vi "svfa_Compute Dual Cross Spectrum Subset.vi"(0 "Windowed signal [X]":waveform(dbl), 1 "processing control":T7(ring), 2 "Spectrum Settings":T10 {"stop frequency" format="%.2f"; "start frequency" format="%.2f"}, 5 "Windowed signal [Y]":waveform(dbl), 7 "window":u16(ring)=1 items=["None "=0, "Hanning"=1, "Hamming"=2, "Blackman-Harris"=3, "Exact Blackman"=4, "Blackman"=5, "Flat Top"=6, "4 Term B-Harris "=7, "7 Term B-Harris"=8, "Low Sidelobe"=9, "Force - Exponential"=10, "Gaussian"=62], 9 "window size":i32, 11 "error in":errorcluster, 12 "averaging parameters":T9={"averaging mode"=enum."No averaging", "weighting mode"=enum."Linear", "number of averages"=10, "linear mode"=enum."Auto restart"}, 13 "spectrum info in":T1={"channel name"="", "description"="", "x-axis units"=0, "spectral info"={"spectrum type"=enum."Power [Magnitude^2]", "linear/dB"=enum."linear", "window"=0, "window size"=0, "FFT size"=0}, "engineering units"=0, "custom label"="", "dB reference [EU]"=0.0, "peak units"=enum."rms", "weighting filter"=0, "spectral density?"=FALSE, "unit label"="", "spectrum skewed?"=FALSE, "complimentary spectrum units"=enum."none"} {"x-axis units" items=["Time (s)"=0, "Frequency-CB (Hz)"=1, "Frequency-CPB (Hz)"=1248, "Frequency-Arbitrary (Hz)"=2357, "Quefrency (s)"=2, "Revolutions (rev)"=3, "Order"=4, "Speed (RPM)"=11, "Speed (rad/s)"=21, "Index"=65535]; "weighting filter" items=["Linear", "A-weighting", "B-weighting", "C-weighting", "ITU-R 468-4", "Dolby", "CCITT", "C-message", "Wb", "Wc", "Wd", "We", "Wf", "Wh", "Wj", "Wk", "Wm", "AES17 20 kHz lowpass", "AES17 40 kHz lowpass", "AES17 20 kHz highpass", "AES17 40 kHz highpass"]; "dB reference [EU]" format="%.2f"; "engineering units" items=["custom..."=0, "V"=1, "A"=21, "C"=30, "pC"=31, "s"=32, "-"=29, "Pa"=2, "N"=20, "g"=3, "m/s^2"=4, "m/s"=5, "m"=6, "mm/s"=12, "mm"=13, "micron/s"=14, "micron"=15, "in/s^2"=7, "in/s"=8, "in"=9, "mil/s"=10, "mil"=11, "rad/s^2"=16, "rad/s"=17, "rad"=18, "deg/s^2"=26, "deg/s"=27, "deg"=28, "RPM"=22, "cycle/s^2"=23, "Hz"=24, "cycle"=25, "strain"=19]; "spectral info"."window" items=["None "=0, "Hanning"=1, "Hamming"=2, "Blackman-Harris"=3, "Exact Blackman"=4, "Blackman"=5, "Flat Top"=6, "4 Term B-Harris "=7, "7 Term B-Harris"=8, "Low Sidelobe"=9, "Force - Exponential"=10, "Gaussian"=62]}) -> (4 "complex spectrum":T8={"f0"=0.0, "df"=1.0, "complex spectrum"=[]} {"complex spectrum" format="%.2f"; "df" format="%.2f"; "f0" format="%.2f"}, 6 "averaging done":bool, 8 "averages completed":dbl format="%.2f", 10 "spectrum info out":T1={"channel name"="", "description"="", "x-axis units"=0, "spectral info"={"spectrum type"=enum."Power [Magnitude^2]", "linear/dB"=enum."linear", "window"=0, "window size"=0, "FFT size"=0}, "engineering units"=0, "custom label"="", "dB reference [EU]"=0.0, "peak units"=enum."rms", "weighting filter"=0, "spectral density?"=FALSE, "unit label"="", "spectrum skewed?"=FALSE, "complimentary spectrum units"=enum."none"} {"x-axis units" items=["Time (s)"=0, "Frequency-CB (Hz)"=1, "Frequency-CPB (Hz)"=1248, "Frequency-Arbitrary (Hz)"=2357, "Quefrency (s)"=2, "Revolutions (rev)"=3, "Order"=4, "Speed (RPM)"=11, "Speed (rad/s)"=21, "Index"=65535]; "weighting filter" items=["Linear", "A-weighting", "B-weighting", "C-weighting", "ITU-R 468-4", "Dolby", "CCITT", "C-message", "Wb", "Wc", "Wd", "We", "Wf", "Wh", "Wj", "Wk", "Wm", "AES17 20 kHz lowpass", "AES17 40 kHz lowpass", "AES17 20 kHz highpass", "AES17 40 kHz highpass"]; "dB reference [EU]" format="%.2f"; "engineering units" items=["custom..."=0, "V"=1, "A"=21, "C"=30, "pC"=31, "s"=32, "-"=29, "Pa"=2, "N"=20, "g"=3, "m/s^2"=4, "m/s"=5, "m"=6, "mm/s"=12, "mm"=13, "micron/s"=14, "micron"=15, "in/s^2"=7, "in/s"=8, "in"=9, "mil/s"=10, "mil"=11, "rad/s^2"=16, "rad/s"=17, "rad"=18, "deg/s^2"=26, "deg/s"=27, "deg"=28, "RPM"=22, "cycle/s^2"=23, "Hz"=24, "cycle"=25, "strain"=19]; "spectral info"."window" items=["None "=0, "Hanning"=1, "Hamming"=2, "Blackman-Harris"=3, "Exact Blackman"=4, "Blackman"=5, "Flat Top"=6, "4 Term B-Harris "=7, "7 Term B-Harris"=8, "Low Sidelobe"=9, "Force - Exponential"=10, "Gaussian"=62]}, 15 "error out":errorcluster)   [LabVIEW 2017]
uses:
  <vilib>/addons/_NISVFA/_Shared subVIs/Controls/svc_Spectrum Info.ctl
  <vilib>/addons/_NISVFA/_Shared subVIs/Controls/svc_X-Axis Units.ctl
  <vilib>/addons/_NISVFA/_Shared subVIs/Controls/svc_Spectrum Type.ctl
  <vilib>/addons/_NISVFA/_Shared subVIs/Controls/svc_Engineering Units Text Ring.ctl
  <vilib>/addons/_NISVFA/_Shared subVIs/Controls/svc_Weighting Filter Text Ring.ctl
  <vilib>/addons/_NISVFA/_Shared subVIs/Controls/svc_Complimentary Spectrum Units.ctl
  <vilib>/addons/_NISVFA/_Shared subVIs/Spectrum Averaging/svfa_Average Spectrum (complex) No State.vi
  <vilib>/addons/_NISVFA/_Shared subVIs/Spectrum Averaging/svfa_Reset Averaging State Info.vi
  <vilib>/addons/_NISVFA/_Shared subVIs/Spectrum Averaging/svfa_Average Array with Avg Checks (complex) No State.vi
  <vilib>/addons/_NISVFA/_Shared subVIs/Spectrum Averaging/svfa_Average Array (complex) No State.vi
  <vilib>/addons/_NISVFA/_Shared subVIs/Spectrum Averaging/svfa_No Average Array (complex).vi
  <vilib>/addons/_NISVFA/_Shared subVIs/Spectrum Averaging/svfa_Average Array (complex).vi
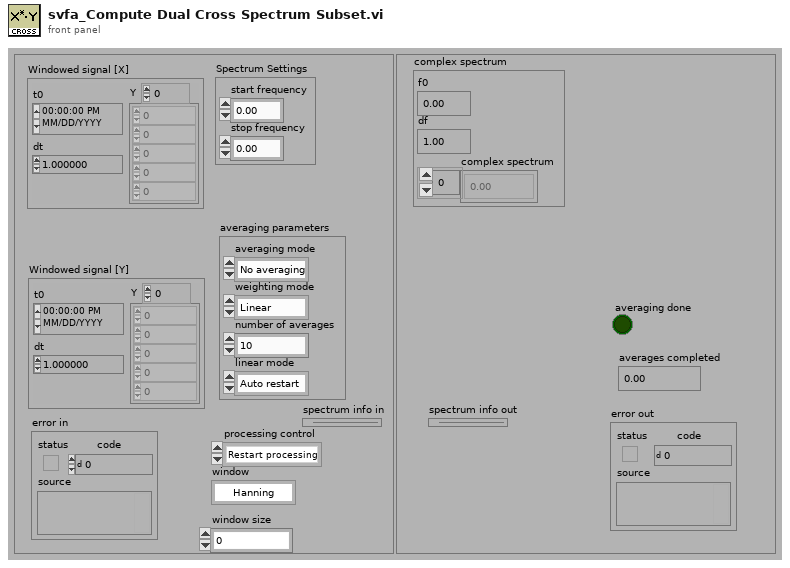
[diagram p1: front panel]
types:
  T1 = typedef "svc_Spectrum Info.ctl" = cluster{"channel name":string, "description":string, "x-axis units":T2, "spectral info":cluster{"spectrum type":T3, "linear/dB":enum16{"linear", "dB"}, "window":u16, "window size":i32, "FFT size":i32}, "engineering units":T4, "custom label":string, "dB reference [EU]":dbl, "peak units":enum16{"rms", "peak", "peak-peak"}, "weighting filter":T5, "spectral density?":bool, "unit label":string, "spectrum skewed?":bool, "complimentary spectrum units":T6}
  T2 = typedef "svc_X-Axis Units.ctl" = u16
  T3 = typedef "svc_Spectrum Type.ctl" = enum16{"FFT Spectrum [complex]", "Amplitude [Magnitude]", "Power [Magnitude^2]", "Cross Spectrum [complex]", "Frequency Response [Complex]"}
  T4 = typedef "svc_Engineering Units Text Ring.ctl" = u16
  T5 = typedef "svc_Weighting Filter Text Ring.ctl" = u16
  T6 = typedef "svc_Complimentary Spectrum Units.ctl" = enum16{"none", "radians", "degrees", "cycles", "imaginary"}
  T7 = enum16{"Restart processing", "Continue processing", "Skip processing"}
  T8 = cluster{"f0":dbl, "df":dbl, "complex spectrum":cdb[]}
  T9 = cluster{"averaging mode":enum16{"No averaging", "Vector averaging", "RMS averaging", "Peak hold"}, "weighting mode":enum16{"Linear", "Exponential"}, "number of averages":u32, "linear mode":enum16{"One shot", "Auto restart"}}
  T10 = cluster{"start frequency":dbl, "stop frequency":dbl}
  T11 = enum16{"No averaging", "Vector averaging", "RMS averaging", "Peak hold"}
  T12 = cluster{"complex spectrum":cluster{"f0":dbl, "df":dbl, "complex spectrum":cdb[]}, "spectrum info":T1}
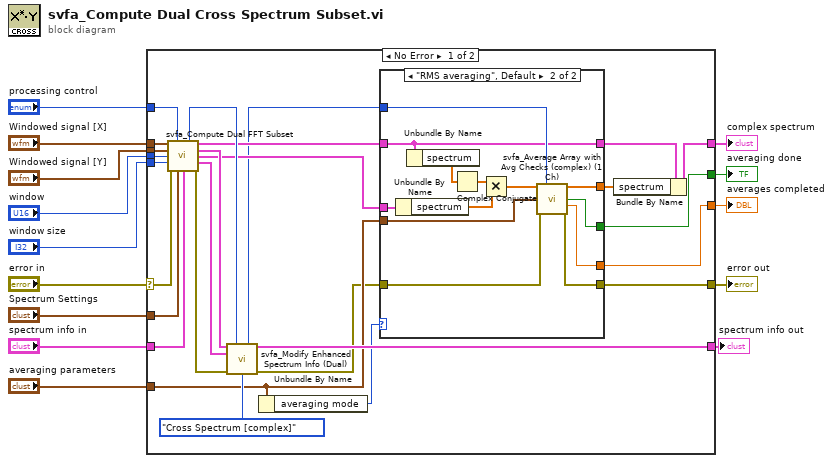
[diagram p0: block diagram]
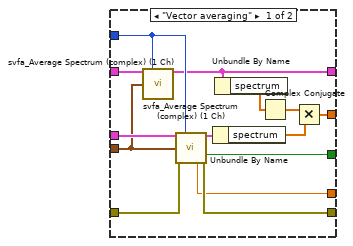
[diagram p2: hidden frame]
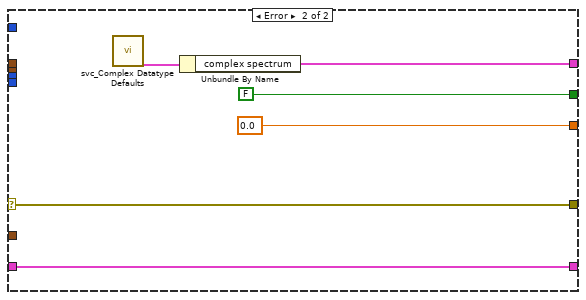
[diagram p3: hidden frame]
diagram:
  n1 = case shown="No Error" "error in" {
    selector: "error in" -> [w38 w72]
    tunnel: [w19 w72] -> w14
    tunnel: "Spectrum Settings" -> [w34 _]
    tunnel: "Windowed signal [Y]" -> [w40 _]
    tunnel: "Windowed signal [X]" -> [w39 _]
    tunnel: "averaging parameters" -> [w17 _]
    tunnel: [w21 0.0 ("averages completed")] -> w9
    tunnel: [w20 FALSE ("averaging done?")] -> w8
    tunnel: [w22 w68] -> w7
    tunnel: "processing control" -> [w30 _]
    tunnel: "window" -> [w33 _]
    tunnel: "window size" -> [w32 _]
    tunnel: [w28 w69] -> w2
    tunnel: "spectrum info in" -> [w27 w69]
    frame No Error {
      n2 = call <vilib>:"svfa_Compute Dual FFT Subset.vi"("Windowed signal [X]"=w39, "processing control"=w30, "Windowed signal [Y]"=w40, "window"=w33, "window size"=w32, "error in (no error)"=w38, "Spectrum Settings"=w34, "spectrum info in"=w27) -> ("dup processing control"=w29:T7, "X FFT spectrum [Vrms]"=w25:cluster{"f0":dbl, "df":dbl, "spectrum":cdb[]}, "spectrum info X"=w37:T1, "Y FFT spectrum [Vrms]"=w24:cluster{"f0":dbl, "df":dbl, "spectrum":cdb[]}, "spectrum info Y"=w36:T1, "error out"=w35:errorcluster)  [unwired: 2 in]
      n3 = call <vilib>:"svfa_Modify Enhanced Spectrum Info (Dual).vi"("spectrum info X"=w37, "processing control"=w29, "spectrum info Y"=w36, "error in (no error)"=w35, "spectrum type"=svc_Spectrum_Type."Cross Spectrum [complex]") -> ("dup processing control"=w18:T7, "spectrum info"=w28:T1, "error out"=w16:errorcluster)  [unwired: 8 in]
      n4 = Unbundle By Name(w17) -> ("averaging mode"=w26:T11)
      n5 = case shown="\"RMS averaging\", Default" w26 {
        tunnel: [w41 w61] -> w21
        tunnel: [w48 w62] -> w20
        tunnel: w17 -> [w47 w59]
        tunnel: w25 -> [w54 w56]
        tunnel: w24 -> [w53 w67]
        tunnel: [w51 w63] -> w23
        tunnel: w16 -> [w43 w58]
        tunnel: [w42 w57] -> w19
        tunnel: w18 -> [w46 w60]
        tunnel: [w44 w56] -> w15
        frame "Vector averaging" {
          n6 = call <vilib>:"svfa_Average Spectrum (complex) (1 Ch).vi"("spectrum"=w54, "processing control"=w46, "averaging parameters"=w47) -> ("spectrum"=w44:cluster{"f0":dbl, "df":dbl, "spectrum":cdb[]})  [unwired: 8 in, 4 out]
          n7 = call <vilib>:"svfa_Average Spectrum (complex) (1 Ch).vi"("spectrum"=w53, "processing control"=w46, "averaging parameters"=w47, "error in (no error)"=w43) -> ("spectrum"=w50:cluster{"f0":dbl, "df":dbl, "spectrum":cdb[]}, "averaging done"=w48:bool, "averages completed"=w41:dbl, "error out"=w42:errorcluster)  [unwired: 7 in, 1 out]
          n8 = Unbundle By Name(w50) -> ("spectrum"=w45:cdb[])
          n9 = Unbundle By Name(w44) -> ("spectrum"=w49:cdb[])
          n10 = Complex Conjugate(1:w49) -> (0:w52:cdb[])
          n11 = Multiply(x=w52, y=w45) -> (x*y=w51:cdb[])
        }
        frame "RMS averaging", Default {
          n12 = Unbundle By Name(w67) -> ("spectrum"=w55:cdb[])
          n13 = Unbundle By Name(w56) -> ("spectrum"=w66:cdb[])
          n14 = Complex Conjugate(1:w66) -> (0:w65:cdb[])
          n15 = Multiply(x=w65, y=w55) -> (x*y=w64:cdb[])
          n16 = call <vilib>:"svfa_Average Array with Avg Checks (complex) (1 Ch).vi"("spectrum"=w64, "processing control"=w60, "averaging parameters"=w59, "error in (no error)"=w58) -> ("average spectrum"=w63:cdb[], "averaging done"=w62:bool, "averages completed"=w61:dbl, "error out"=w57:errorcluster)  [unwired: 7 in, 1 out]
        }
      }
      n17 = Bundle By Name(cluster=w15, "spectrum"=w23) -> (w22:cluster{"f0":dbl, "df":dbl, "spectrum":cdb[]})
    }
    frame Error {
      n18 = call <vilib>:"svc_Complex Datatype Defaults.vi"() -> ("complex spectrum"=w70:T12)  [unwired: 11 in, 8 out]
      n19 = Unbundle By Name(w70) -> ("complex spectrum"=w68:T8)
    }
  }
  "error out" <- w14
  "averages completed" <- w9
  "averaging done" <- w8
  "complex spectrum" <- w7
  "spectrum info out" <- w2
